vi "ReadDeviceID Example.vi"() -> ()   [LabVIEW 2012]
uses:
  BrooksDLL.dll
panel:
  in  "Drop Type":i32(ring)=1 items=["Single Drop", "Multi-Drop"]
  out "S2 String":string
  out "S1 String":string
  out "S2":u8 format="%.0x"
  out "S1":u8 format="%.0x"
  out "Function Output Comment":string
  in  "IDS":u8 format="%.0x"
  in  "IDL":u8 format="%.0x"
  in  "IDM":u8 format="%.0x"
  in  "IDH":u8 format="%.0x"
  out "output param":i32
  # "These four values are displayed as hexadecimal, and hexadecimal notation is used in the subsequent examples"
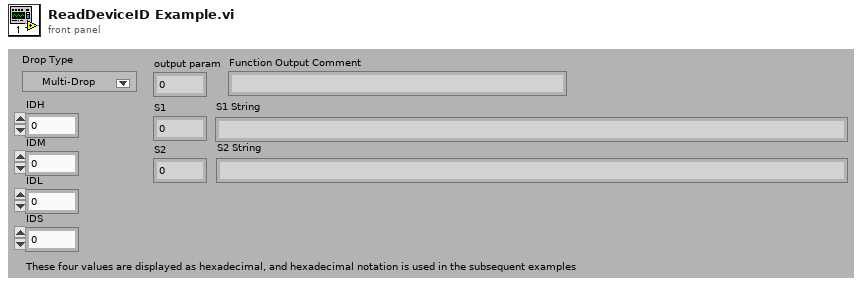
[diagram p1: front panel]
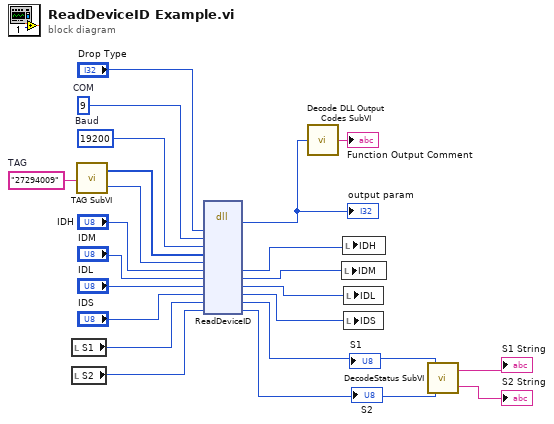
[diagram p0: block diagram]
diagram:
  w18 = "27294009"  # TAG
  w17 = 19200  # Baud
  w16 = 9  # COM
  n1 = local read "S1"() -> (w13:u8)
  n2 = local read "S2"() -> (w14:u8)
  n3 = call "TAG SubVI.vi"("TAG String"=w18) -> ("TAG"=w2:u8[], "Length"=w1:i32)
  n4 = dll-call lib="C:/Users/Sylvain/Downloads/164j027_ac/S Protocol/BrooksDLL.dll" fn="ReadDeviceID"("DropType"="Drop Type", "COM"=w16, "Baud"=w17, "TAG"=w2, "Length"=w1, "IDH"="IDH", "IDM"="IDM", "IDL"="IDL", "IDS"="IDS", "S1"=w13, "S2"=w14) -> (w22:i32, "IDH"=w3:u8, "IDM"=w4:u8, "IDL"=w5:u8, "IDS"=w6:u8, "S1"=w7:u8, "S2"=w8:u8)  [unwired: 8 in, 2 out]
  "output param" <- w22
  "S1" <- w7
  "S2" <- w8
  n5 = call "Decode DLL Output Codes SubVI.vi"("Numeric"=w22) -> ("Function Output Comment"=→"Function Output Comment":string)
  n6 = local write "IDM"(w4) -> ()
  n7 = local write "IDH"(w3) -> ()
  n8 = local write "IDL"(w5) -> ()
  n9 = local write "IDS"(w6) -> ()
  n10 = call "DecodeStatus SubVI.vi"("S2"=w8, "S1"=w7) -> ("S2 String"=→"S2 String":string, "S1 String"=→"S1 String":string)
